vi "Save Test Information.vi"(8 "error in (no error)":errorcluster, 10 "Test Information":T1, 11 "TestMonitor in":refnum<class "TestMonitor.lvclass">) -> (0 "error out":errorcluster, 3 "TestMonitor out":refnum<class "TestMonitor.lvclass">)   [LabVIEW 2018, in "TestMonitor.lvclass"]
doc: "This VI will save the Test Information to the permanent report"
uses:
  TestMonitor.lvclass
  Report Information/Test Information.ctl
  TestMonitor.lvclass/TestMonitor.ctl
  <vilib>/Skyline/TestMonitor/Test Result/Update Test Result (Single).vi
  <vilib>/Skyline/TestMonitor/Test Result/NI SystemLink Test Result.lvclass
  Report Information/Report Information.lvclass
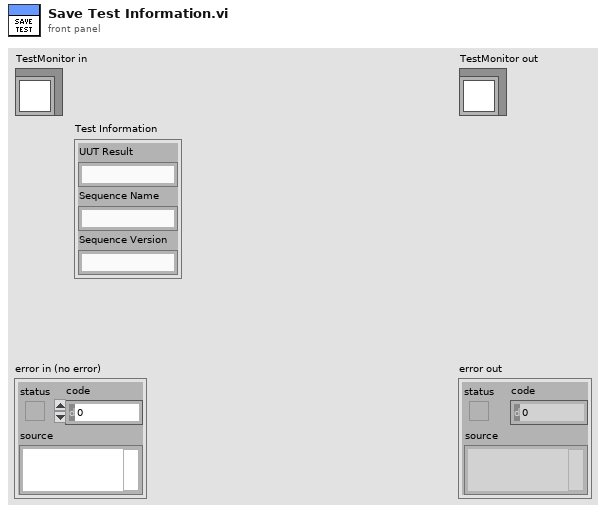
[diagram p1: front panel]
types:
  T1 = typedef "Report Information.lvclass/Test Information.ctl" = cluster{"UUT Result":string, "Sequence Name":string, "Sequence Version":string}
  T2 = typedef "NI Skyline Utilities.lvlib/Property.ctl" = cluster{"key":string, "value":string}
  T3 = typedef "NI SystemLink Test Monitor.lvlib/Status Type.ctl" = enum16{"Failed", "Passed", "Looping", "Skipped", "Custom", "Done", "Running", "Waiting", "Terminated", "Errored", "Timed Out", "None"}
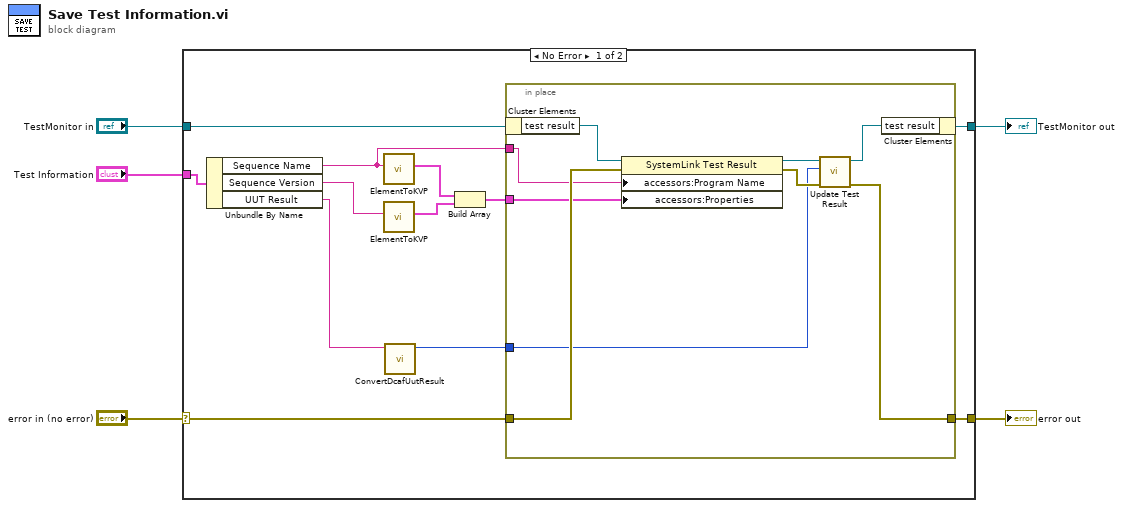
[diagram p0: block diagram]
diagram:
  n1 = case shown="No Error" "error in (no error)" {
    selector: "error in (no error)" -> [w15 w28]
    tunnel: [w14 w28] -> w5
    tunnel: [w12 w27] -> w3
    tunnel: "TestMonitor in" -> [w16 w27]
    tunnel: "Test Information" -> [w17 _]
    frame No Error {
      n2 = Unbundle By Name(w17) -> ("Sequence Name"=w6:string, "Sequence Version"=w9:string, "UUT Result"=w11:string)
      n3 = call "ElementToKVP.vi"("Element"=w6) -> ("KVP"=w8:T2)  [unwired: 9 in, 1 out]
      n4 = call "ElementToKVP.vi"("Element"=w9) -> ("KVP"=w7:T2)  [unwired: 9 in, 1 out]
      n5 = call "ConvertDcafUutResult.vi"("UUT Result"=w11) -> ("Systemlink Status"=w10:T3)  [unwired: 10 in]
      n6 = Build Array(w8, w7) -> (w13:T2[])
      n7 = in-place {
        in-place-border: w15 -> [w24]
        in-place-border: [w21] -> w14
        in-place-border: w13 -> [w19]
        in-place-border: w10 -> [w20]
        in-place-border: w6 -> [w18]
        n8 = in-place-cluster #1(w16) -> ("test result"=w26:refnum<class "NI SystemLink Test Result.lvclass">)
        n9 = property class="SystemLink Test Result"(reference=w26, error in=w24, "accessors:Program Name"=w18, "accessors:Properties"=w19) -> (reference out=w25:refnum<class "NI SystemLink Test Result.lvclass">, error out=w22:errorcluster)
        n10 = call-poly <vilib>:"Update Test Result.vi"("error in (no error)"=w22, "status type"=w20, "test result in"=w25) -> ("error out"=w21:errorcluster, "test result out"=w23:refnum<class "NI SystemLink Test Result.lvclass">)  [unwired: 7 in]
        n11 = in-place-cluster #1("test result"=w23) -> (w12:refnum<class "TestMonitor.lvclass">)
      }
    }
    frame Error {
    }
  }
  "error out" <- w5
  "TestMonitor out" <- w3
